vi "test_libssh2_channel_write.vi"() -> ()   [LabVIEW 2017, in "integration_tests.lvlib"]
uses:
  integration_tests.lvlib
  libssh2/libssh2_channel_open_ex.vi
  libssh2/libssh2_channel_process_startup.vi
  libssh2/libssh2_channel_write_ex.vi
  support/support.lvlib
  libssh2/libssh2.lvlib
  <vilib>/PNR/Transparent Assertions/Transparent Assertions/Transparent Assertions.lvlib
panel:
  out "error out":errorcluster
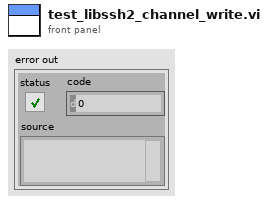
[diagram p1: front panel]
types:
  T1 = typedef "libssh2.lvlib/Session Refnum.ctl" = refnum<k1>
  T2 = typedef "libssh2.lvlib/Channel Refnum.ctl" = refnum<k1>
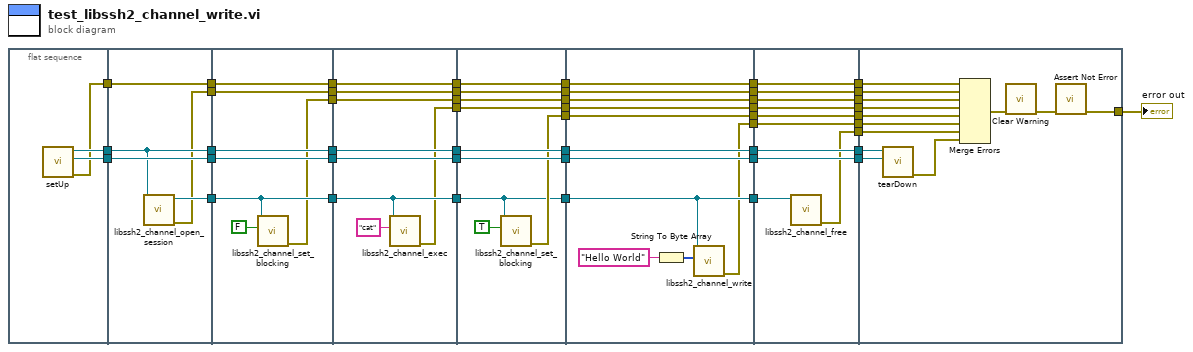
[diagram p0: block diagram]
diagram:
  n1 = flat-sequence {
    tunnel: [w51] -> w48
    tunnel: [w50] -> w47
    tunnel: [w49] -> w46
    tunnel: w48 -> [w55]
    tunnel: w47 -> [w56]
    tunnel: [w55] -> w38
    tunnel: [w56] -> w36
    tunnel: [w54] -> w30
    tunnel: w46 -> [w53]
    tunnel: [w53] -> w34
    tunnel: [w52] -> w32
    tunnel: w38 -> [w63]
    tunnel: [w63] -> w37
    tunnel: w36 -> [w62]
    tunnel: [w62] -> w35
    tunnel: w34 -> [w61]
    tunnel: [w61] -> w33
    tunnel: w32 -> [w60]
    tunnel: [w60] -> w31
    tunnel: w30 -> [w59]
    tunnel: [w59] -> w29
    tunnel: [w57] -> w28
    tunnel: w37 -> [w71]
    tunnel: [w71] -> w26
    tunnel: w35 -> [w70]
    tunnel: [w70] -> w24
    tunnel: w33 -> [w69]
    tunnel: [w69] -> w22
    tunnel: w31 -> [w68]
    tunnel: [w68] -> w20
    tunnel: w29 -> [w67]
    tunnel: [w67] -> w18
    tunnel: [w65] -> w16
    tunnel: w28 -> [w64]
    tunnel: [w64] -> w14
    tunnel: w26 -> [w80]
    tunnel: [w80] -> w25
    tunnel: w24 -> [w79]
    tunnel: [w79] -> w23
    tunnel: w22 -> [w78]
    tunnel: [w78] -> w21
    tunnel: w20 -> [w77]
    tunnel: [w77] -> w19
    tunnel: w18 -> [w72]
    tunnel: [w72] -> w17
    tunnel: w16 -> [w76]
    tunnel: [w76] -> w15
    tunnel: w14 -> [w75]
    tunnel: [w75] -> w13
    tunnel: [w73] -> w12
    tunnel: w25 -> [w91]
    tunnel: [w91] -> w10
    tunnel: w23 -> [w90]
    tunnel: [w90] -> w9
    tunnel: w21 -> [w89]
    tunnel: [w89] -> w8
    tunnel: w19 -> [w88]
    tunnel: [w88] -> w7
    tunnel: w17 -> [w87]
    tunnel: [w87] -> w6
    tunnel: w15 -> [w86]
    tunnel: [w86] -> w5
    tunnel: w13 -> [w85]
    tunnel: [w85] -> w4
    tunnel: w12 -> [w84]
    tunnel: [w84] -> w3
    tunnel: [w81] -> w2
    tunnel: w10 -> [w101]
    tunnel: w9 -> [w100]
    tunnel: [w101] -> w45
    tunnel: [w100] -> w44
    tunnel: [w99] -> w43
    tunnel: w8 -> [w98]
    tunnel: [w98] -> w42
    tunnel: w7 -> [w97]
    tunnel: [w97] -> w41
    tunnel: w6 -> [w96]
    tunnel: w5 -> [w95]
    tunnel: [w95] -> w39
    tunnel: w4 -> [w94]
    tunnel: [w94] -> w27
    tunnel: w3 -> [w93]
    tunnel: [w93] -> w11
    tunnel: w2 -> [w92]
    tunnel: [w92] -> w1
    tunnel: w45 -> [w114]
    tunnel: w44 -> [w113]
    tunnel: [w112] -> w40
    tunnel: w43 -> [w110]
    tunnel: w42 -> [w109]
    tunnel: w41 -> [w107]
    tunnel: w39 -> [w106]
    tunnel: w27 -> [w105]
    tunnel: w11 -> [w104]
    tunnel: w1 -> [w103]
    frame #0 {
      n2 = call "setUp.vi"() -> ("error out"=w49:errorcluster, "connection ID"=w50:refnum<k5>, "session"=w51:T1)  [unwired: 9 in]
    }
    frame #1 {
      n3 = call "libssh2_channel_open_session.vi"("session"=w55) -> ("error out"=w52:errorcluster, "channel"=w54:T2)  [unwired: 9 in]
    }
    frame #2 {
      n4 = call "libssh2_channel_set_blocking.vi"("blocking"=FALSE, "channel"=w59) -> ("error out"=w57:errorcluster)  [unwired: 9 in]
    }
    frame #3 {
      n5 = call "libssh2_channel_exec.vi"("command"="cat", "channel"=w67) -> ("error out"=w65:errorcluster)  [unwired: 9 in]
    }
    frame #4 {
      n6 = call "libssh2_channel_set_blocking.vi"("blocking"=TRUE, "channel"=w72) -> ("error out"=w73:errorcluster)  [unwired: 9 in]
    }
    frame #5 {
      n7 = String To Byte Array(string="Hello World") -> (unsigned byte array=w83:u8[])
      n8 = call "libssh2_channel_write.vi"("buffer"=w83, "channel"=w87) -> ("error out"=w81:errorcluster)  [unwired: 8 in, 1 out]
    }
    frame #6 {
      n9 = call "libssh2_channel_free.vi"("channel"=w96) -> ("error out"=w99:errorcluster)  [unwired: 10 in]
    }
    frame #7 {
      n10 = call "tearDown.vi"("connection ID"=w113, "session"=w114) -> ("error out"=w111:errorcluster)  [unwired: 9 in]
      n11 = Merge Errors(w109, w107, w105, w106, w104, w103, w110, w111) -> (w108:errorcluster)
      n12 = call "Clear Warning.vi"("error in (no error)"=w108) -> ("error out"=w102:errorcluster)  [unwired: 10 in]
      n13 = call <vilib>:"Assert Not Error.vi"("error in (no error)"=w102) -> ("error out"=w112:errorcluster)  [unwired: 10 in]
    }
  }
  "error out" <- w40
